vi "PSOCE_Protocol_Original.vi"(0 "y_center":dbl, 1 "n_lines":i32=50, 2 "n frames":i32=20, 3 "3D frame":i32=2, 5 "y_span":dbl, 7 "galvo phase":i32, 9 "x_center":dbl, 11 "x_span":dbl=5.0, 12 "flyback_lines":i32=4, 13 "Custom trig.":T1={"n_frames to c. trig"=1, "custom trig length (frames)"=1, "n_frames between c. trig"=1, "n_custom trigger"=1}, 14 "B_frame_rep":i32) -> (4 "x_data":dbl[](graph), 6 "y_data":dbl[](graph), 8 "trigger out":u32[](graph), 10 "custom trig out":u32[](graph), 15 "Overall Frames":i32)   [LabVIEW 2024]
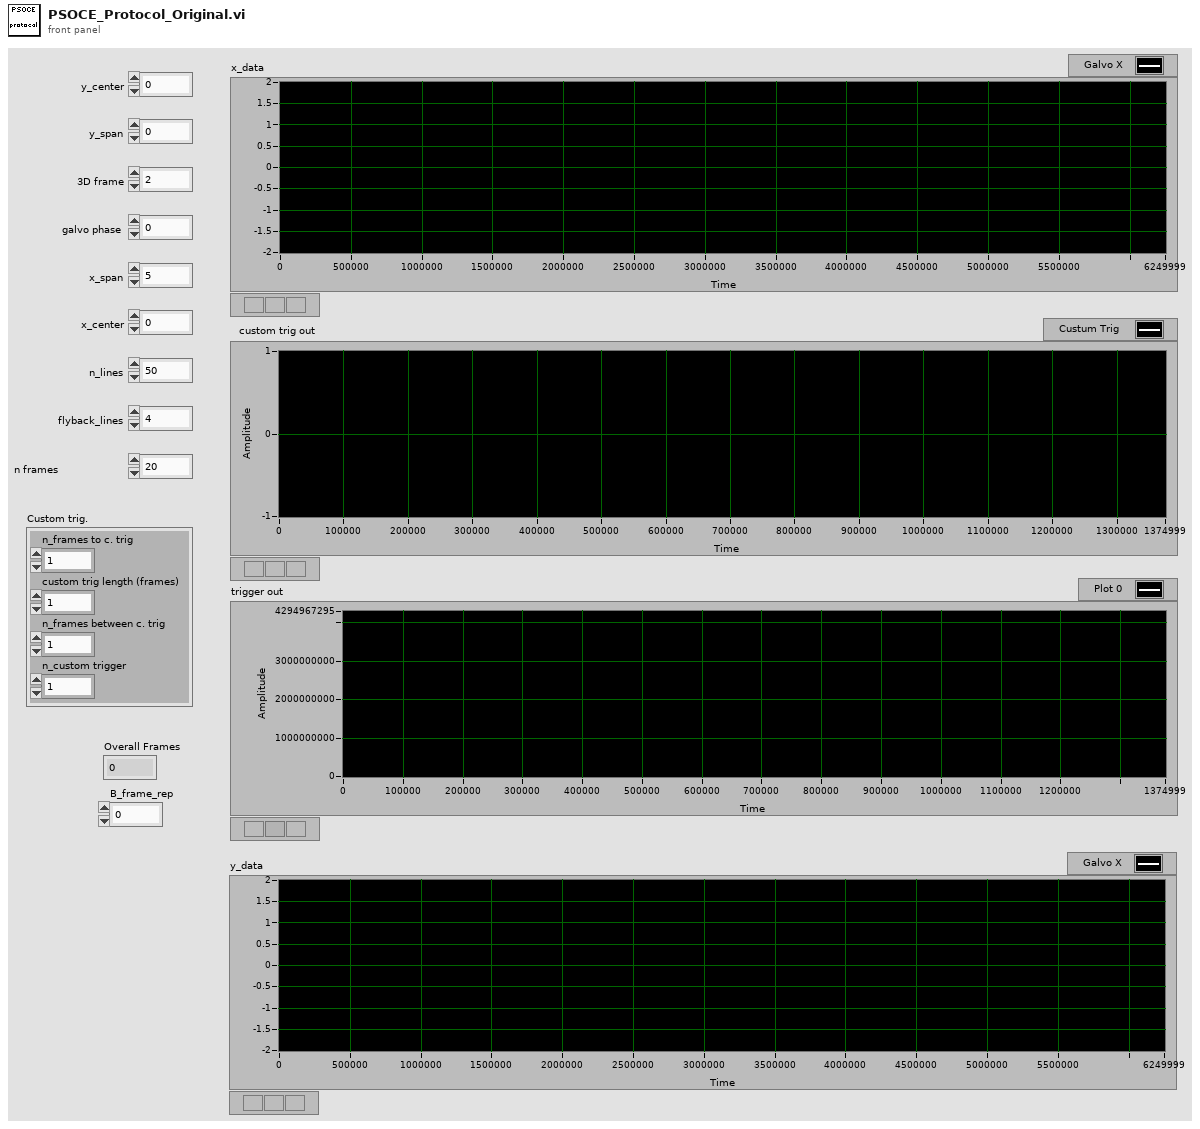
[diagram p1: front panel]
types:
  T1 = cluster{"n_frames to c. trig":i32, "custom trig length (frames)":i32, "n_frames between c. trig":i32, "n_custom trigger":i32}
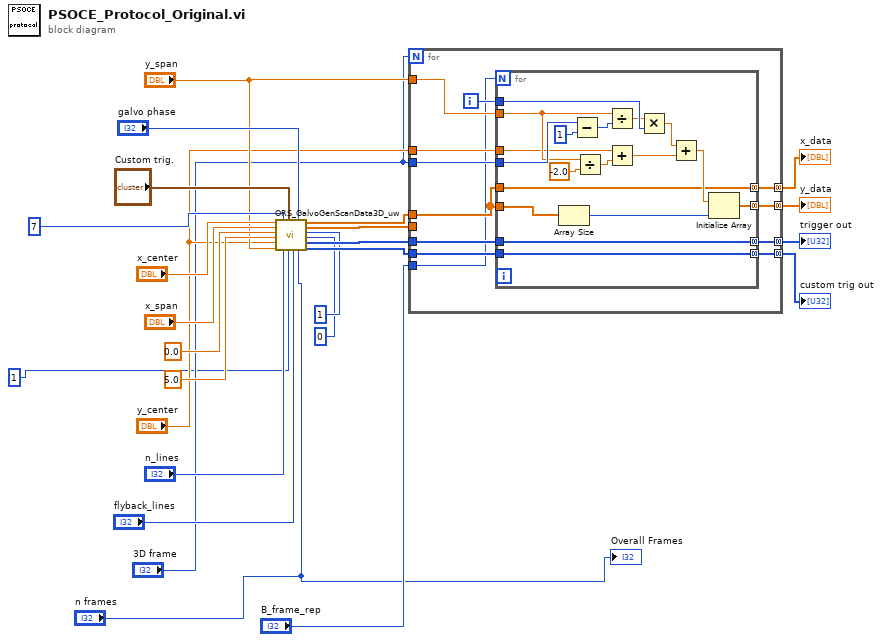
[diagram p0: block diagram]
diagram:
  n1 = call "ORS_GalvoGenScanData3D_uw.vi"("x_center"="x_center", "x_span"="x_span", "offset"=0.0, "span-factor"=5.0, "y_center"="y_center", "y_span"="y_span", "mode"=7, "n_lines"="n_lines", "Custom trig."="Custom trig.", "n_frames same y pos"=u32 1 ("n_3D scans"), "flyback_lines"="flyback_lines", "galvo phase"="galvo phase", "n_frames"="n frames", "n_3D scans"=u32 1, "flyback frames"=u16 0) -> ("x_data"=w18:dbl[], "y_data"=w13:dbl[], "trigger out"=w14:u32[], "custom trig out"=w16:u32[])  [unwired: 1 out]
  n2 = for {
    N: "3D frame" -> [_]
    tunnel: w18 -> [w31]
    tunnel: [w28] -> w17 mode=concatenating
    tunnel: w16 -> [w27]
    tunnel: [w30] -> w15 mode=concatenating
    tunnel: w14 -> [w29]
    tunnel: w13 -> [_]
    tunnel: "3D frame" -> [w37]
    tunnel: "y_span" -> [w35]
    tunnel: "y_center" -> [w34]
    tunnel: [w33] -> w6 mode=concatenating
    tunnel: [w32] -> w4 mode=concatenating
    tunnel: "B_frame_rep" -> [w26]
    i -> [w36]
    n3 = for {
      N: w26 -> [_]
      tunnel: w37 -> [w53]
      tunnel: w36 -> [w50]
      tunnel: w35 -> [w48]
      tunnel: w34 -> [w45]
      tunnel: [w42] -> w33 mode=concatenating
      tunnel: w31 -> [w41]
      tunnel: [w40] -> w32 mode=concatenating
      tunnel: w31 -> [w40]
      tunnel: [w39] -> w30 mode=concatenating
      tunnel: w29 -> [w39]
      tunnel: [w38] -> w28 mode=concatenating
      tunnel: w27 -> [w38]
      n4 = Array Size(array=w41) -> (size(s)=w55:i32)
      n5 = Subtract(x=w53, y=1) -> (x-y=w54:i32)
      n6 = Divide(x=w48, y=-2.0) -> (x/y=w46:dbl)
      n7 = Divide(x=w48, y=w54) -> (x/y=w49:dbl)
      n8 = Add(x=w45, y=w46) -> (x+y=w44:dbl)
      n9 = Multiply(x=w49, y=w50) -> (x*y=w51:dbl)
      n10 = Add(x=w51, y=w44) -> (x+y=w43:dbl)
      n11 = Initialize Array(w43, w55) -> (w42:dbl[])
    }
  }
  "x_data" <- w4
  "custom trig out" <- w17
  "trigger out" <- w15
  "y_data" <- w6
  "Overall Frames" <- "n frames"
